vi "CoerceSpikes.vi"(10 "spikyData":dbl[](array[numeric]), 11 "+/-Nsigma":dbl=3.0) -> (0 "spikesReplaced":i16, 1 "variance":dbl, 2 "mean":dbl, 3 "deSpikedData":dbl[](array[numeric]))   [LabVIEW 2016]
doc: "Takes an input signal and replaces any points in it more than N sigma from the mean with the mean"
uses:
  <vilib>/Analysis/NI_AALBase.lvlib
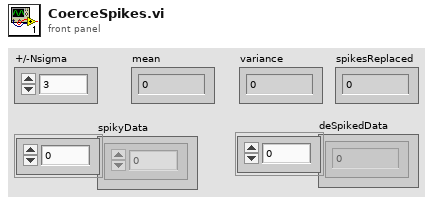
[diagram p1: front panel]
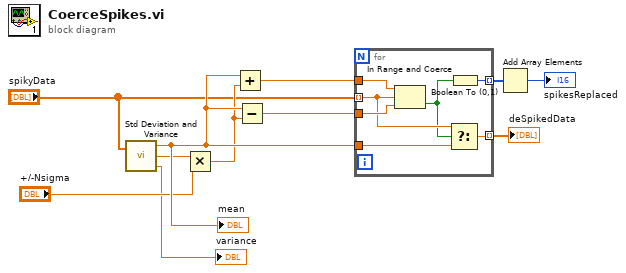
[diagram p0: block diagram]
diagram:
  n1 = call <vilib>:"Std Deviation and Variance.vi"("X"="spikyData") -> ("mean"=w10:dbl, "standard deviation"=w6:dbl, "variance"=→"variance":dbl)  [unwired: 1 in]
  "mean" <- w10
  n2 = Multiply(x=w6, y="+/-Nsigma") -> (x*y=w8:dbl)
  n3 = Add(x=w10, y=w8) -> (x+y=w5:dbl)
  n4 = Subtract(x=w10, y=w8) -> (x-y=w9:dbl)
  n5 = for {
    tunnel: "spikyData" -> [w16] mode=indexing
    tunnel: w5 -> [w18]
    tunnel: w9 -> [w17]
    tunnel: w10 -> [w15]
    tunnel: [w14] -> w11 mode=indexing
    tunnel: [w12] -> w2 mode=indexing
    n6 = In Range and Coerce(upper limit=w18, x=w16, lower limit=w17) -> (In Range?=w13:bool)  [unwired: 1 out]
    n7 = Select(t=w16, s=w13, f=w15) -> (s? t:f=w14:dbl)
    n8 = Boolean To (0,1)(Boolean=w13) -> (0, 1=w12:i16)
  }
  "deSpikedData" <- w11
  n9 = Add Array Elements(numeric array=w2) -> (sum=→"spikesReplaced":i16)
